vi "BRig_Host_comm_tcp_readAccumParse_replaceInvalidChar.vi"(11 "input_string":string) -> (2 "output_stringSize":i32, 3 "output_string":string)   [LabVIEW 2014]
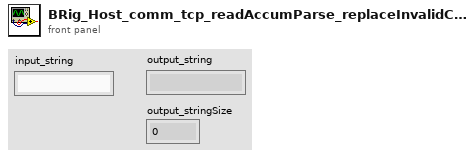
[diagram p1: front panel]
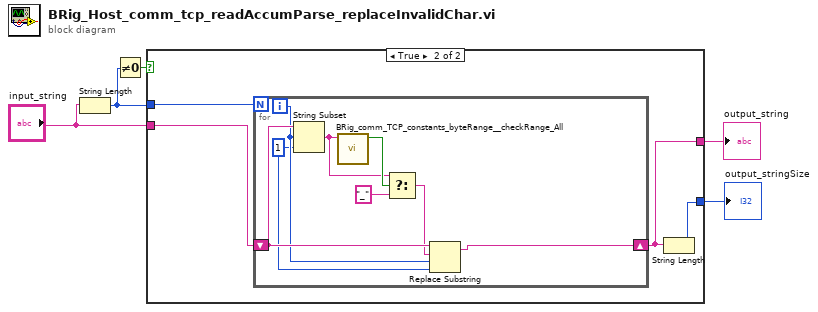
[diagram p0: block diagram]
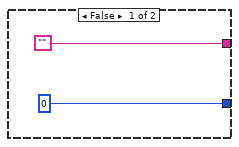
[diagram p2: hidden frame]
diagram:
  n1 = String Length(string="input_string") -> (length=w5:i32)
  n2 = Not Equal To 0?(x=w5) -> (x != 0?=w4:bool)
  n3 = case shown="True" w4 {
    tunnel: w5 -> [_ w11]
    tunnel: "input_string" -> [_ w8]
    tunnel: ["" w9] -> w2
    tunnel: [0 w10] -> w1
    frame False {
    }
    frame True {
      n4 = for {
        N: w11 -> [_]
        shift-right: [w12] -> w9
        shift-left: w8 -> [w16]
        i -> [w14]
        w13 = 1 ("length (rest)")
        n5 = String Subset(string=w16, offset (0)=w14, length (rest)=w13) -> (substring=w18:string)
        n6 = call "BRig_comm_TCP_constants_byteRange__checkRange_All.vi"("input_char"=w18) -> ("output_inRange"=w19:bool)  [unwired: 10 in]
        n7 = Select(t=w18, s=w19, f="_") -> (s? t:f=w15:string)
        n8 = Replace Substring(2:w13, 3:w14, 4:w15, 5:w16) -> (1:w12:string)  [unwired: 1 out]
      }
      n9 = String Length(string=w9) -> (length=w10:i32)
    }
  }
  "output_string" <- w2
  "output_stringSize" <- w1
